vi "libssh2_session_free.vi"(8 "error in (no error)":errorcluster, 11 "session":T1) -> (0 "error out":errorcluster)   [LabVIEW 2013, in "libssh2.lvlib"]
doc: "Frees all resources associated with a session instance."
uses:
  libssh2.lvlib
  Session Refnum.ctl
  Global Settings.vi
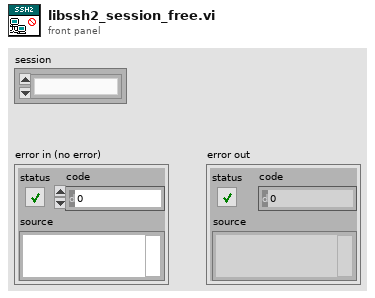
[diagram p1: front panel]
types:
  T1 = typedef "libssh2.lvlib/Session Refnum.ctl" = refnum<k1>
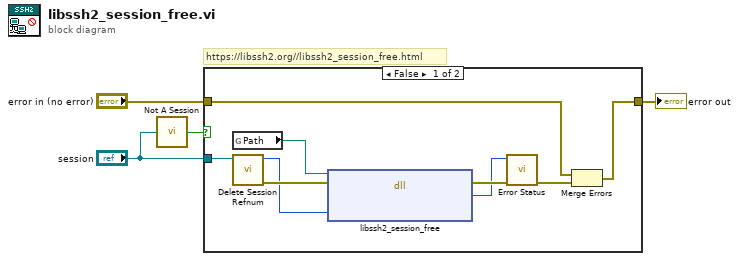
[diagram p0: block diagram]
diagram:
  # "https://libssh2.org//libssh2_session_free.html"
  n1 = call "Not A Session.vi"("session"="session") -> ("Not a Session?"=w1:bool)
  n2 = case shown="False" w1 {
    tunnel: [w9 w14] -> w4
    tunnel: "error in (no error)" -> [w8 w14]
    tunnel: "session" -> [w10 _]
    frame False {
      n3 = global read "Global Settings.vi" "Path"() -> (w7:path)
      n4 = call "Delete Session Refnum.vi"("session"=w10) -> ("error out"=w12:errorcluster, "LIBSSH2_SESSION*"=w11:u64)  [unwired: 9 in]
      n5 = dll-call lib="C:/Users/pasca/source/repos/libssh2-labview/libssh2/libssh2**.*" fn="libssh2_session_free"(path in=w7, error in=w12, "session"=w11) -> (error out=w13:errorcluster, "return value"=w5:i32)  [unwired: 2 in, 1 out]
      n6 = call "Error Status.vi"("error in (no error)"=w13, "return value"=w5) -> ("error out"=w6:errorcluster)  [unwired: 8 in, 1 out]
      n7 = Merge Errors(w8, w6) -> (w9:errorcluster)
    }
    frame True {
    }
  }
  "error out" <- w4
